vi "FRCts20_Backend_INI_Read_Revision.vi"(8 "error in (no error)":errorcluster, 11 "INI Controller in":refnum<class "FRCts20_Backend_INI Controller.lvclass">) -> (0 "error out":errorcluster, 2 "Revision":T1, 3 "INI Controller out":refnum<class "FRCts20_Backend_INI Controller.lvclass">)   [LabVIEW 2013, in "FRCts20_Backend_Engine.lvlib" / "FRCts20_Backend_INI Controller.lvclass"]
uses:
  FRCts20_Backend_INI Controller.lvclass
  FRCts20_Backend_INI_Revision.ctl
  FRCts20_Backend_INI Controller.lvclass/FRCts20_Backend_INI Controller.ctl
  <vilib>/Utility/config.llb/Read Key (String).vi
  <vilib>/Utility/config.llb/NI_LVConfig.lvlib
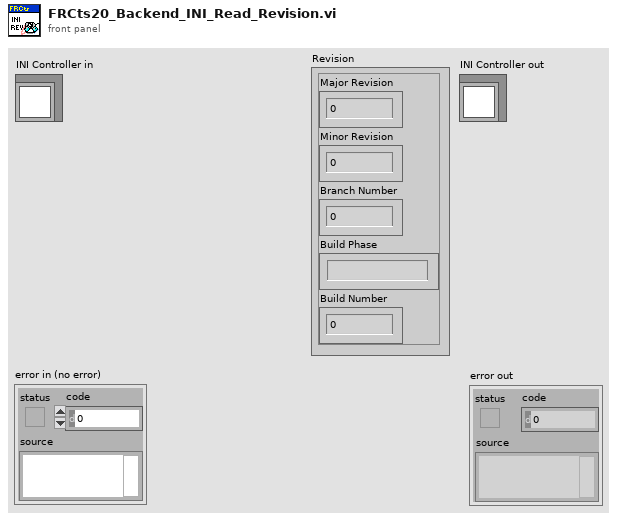
[diagram p1: front panel]
types:
  T1 = typedef "FRCts20_Backend_Engine.lvlib/FRCts20_Backend_INI Controller.lvclass/FRCts20_Backend_INI_Revision.ctl" = cluster{"Major Revision":i32, "Minor Revision":i32, "Branch Number":i32, "Build Phase":string, "Build Number":i32}
  T2 = typedef "NI_LVConfig.lvlib/Config Data RefNum.ctl" = refnum<k1>
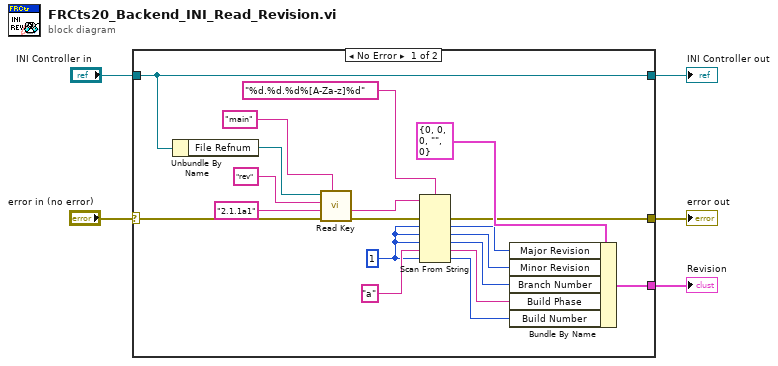
[diagram p0: block diagram]
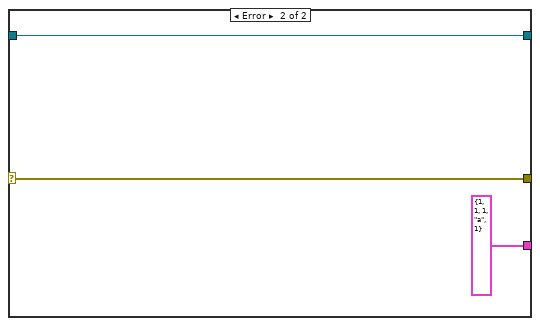
[diagram p2: hidden frame]
diagram:
  n1 = case shown="No Error" "error in (no error)" {
    selector: "error in (no error)" -> [w22 w26]
    tunnel: [w6 w26] -> w4
    tunnel: [w24 w27] -> w2
    tunnel: "INI Controller in" -> [w24 w27]
    tunnel: [w7 T1 {"Major Revision"=1, "Minor Revision"=1, "Branch Number"=1, "Build Phase"="a", "Build Number"=1} ("Cluster")] -> w1
    frame No Error {
      w12 = 1 ("default value 5")
      n2 = Unbundle By Name(w24) -> ("File Refnum"=w23:T2)
      n3 = call-poly <vilib>:"Read Key.vi"("section"="main", "error in (no error)"=w22, "default value"="2.1.1a1", "key"="rev", "refnum"=w23) -> ("error out"=w17:errorcluster, "value"=w18:string)  [unwired: 3 in, 2 out]
      n4 = Scan From String(format string="%d.%d.%d%[A-Za-z]%d", input string=w18, error in=w17, default 1=w12, default 2=w12, default 3=w12, default 4="a" ("default value 4"), default 5=w12) -> (error out=w6:errorcluster, output 1=w8:i32, output 2=w9:i32, output 3=w10:i32, output 4=w14:string, output 5=w11:i32)  [unwired: 1 in, 2 out]
      n5 = Bundle By Name(cluster=T1 {"Major Revision"=0, "Minor Revision"=0, "Branch Number"=0, "Build Phase"="", "Build Number"=0} ("Cluster"), "Major Revision"=w8, "Minor Revision"=w9, "Branch Number"=w10, "Build Phase"=w14, "Build Number"=w11) -> (w7:T1)
    }
    frame Error {
    }
  }
  "error out" <- w4
  "INI Controller out" <- w2
  "Revision" <- w1
